vi "DDVL Quit or Abort VI.vi"(0 "VI Ref":refnum<vi>, 2 "Abort VI?":bool, 11 "Error In":errorcluster) -> (8 "Close Command Successful?":bool)   [LabVIEW 2020]
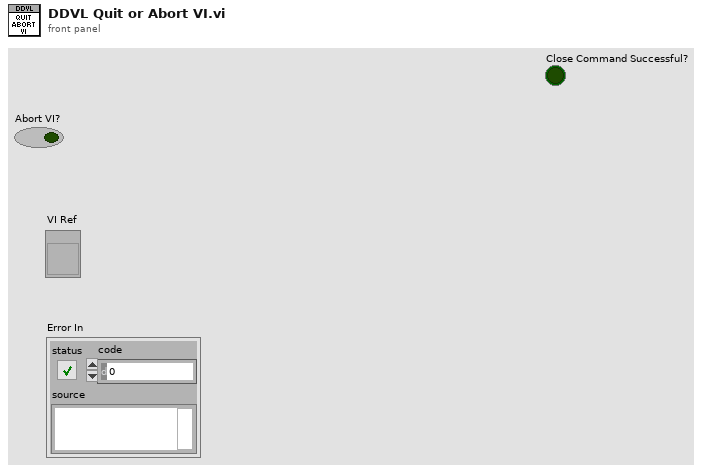
[diagram p1: front panel]
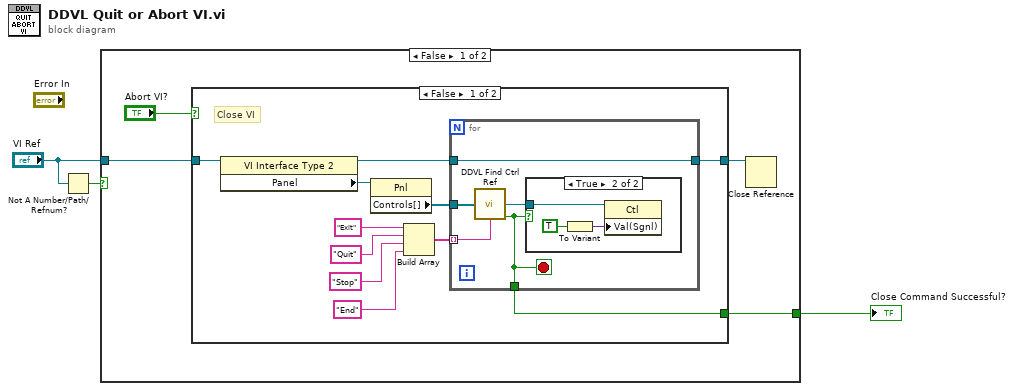
[diagram p0: block diagram]
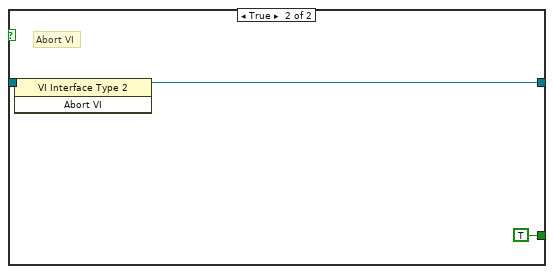
[diagram p3: hidden frame]
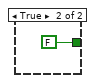
[diagram p4: hidden frame]
diagram:
  n1 = Not A Number/Path/Refnum?(number/path/refnum="VI Ref") -> (NaN/Path/Refnum?=w1:bool)
  n2 = case shown="False" w1 {
    tunnel: "VI Ref" -> [w6 _]
    tunnel: [w4 FALSE] -> w3
    frame False {
      n3 = case shown="False" "Abort VI?" {
        tunnel: w6 -> [w18 w29]
        tunnel: [w10 w28] -> w5
        tunnel: [w8 TRUE ("Control Found?")] -> w4
        frame False {
          # "Close VI"
          n4 = property class="VI Interface Type 2"(reference=w18) -> (reference out=w11:refnum<vi>, "Panel"=w17:refnum<vi>)  [unwired: 1 in, 1 out]
          n5 = property class="Pnl"(reference=w17) -> ("Controls[]"=w16:refnum<vi>[])  [unwired: 1 in, 2 out]
          n6 = Build Array("Exit" ("Control Label"), "Quit" ("Control Label"), "Stop" ("Control Label"), "End" ("Control Label")) -> (w12:string[])
          n7 = for {
            tunnel: w16 -> [w23]
            tunnel: w12 -> [w21] mode=indexing
            tunnel: w11 -> [w20]
            tunnel: [w20] -> w10
            tunnel: [w19] -> w8
            stop <- w19 stop-if-true
            n8 = call "DDVL Find Ctrl Ref.vi"("Control Array"=w23, "Control Label"=w21) -> ("Control Ref"=w22:refnum<vi>, "Control Found?"=w19:bool)  [unwired: 12 in]
            n9 = case shown="True" w19 {
              tunnel: w22 -> [_ w26]
              frame False {
              }
              frame True {
                n10 = To Variant(anything=TRUE) -> (Variant=w25:variant)
                n11 = property class="Ctl"(reference=w26, "Val(Sgnl)"=w25) -> ()  [unwired: 1 in, 2 out]
              }
            }
          }
        }
        frame True {
          # "Abort VI"
          n12 = invoke class="VI Interface Type 2" method="Abort VI"(reference=w29) -> (reference out=w28:refnum<vi>)  [unwired: 2 in, 2 out]
        }
      }
      n13 = Close Reference(reference=w5) -> ()  [unwired: 1 in, 1 out]
    }
    frame True {
    }
  }
  "Close Command Successful?" <- w3
